vi "Finish.vi"   [LabVIEW 2014]
doc: "This VI is called just before exiting. It is expected to close I/O refnum, save collected data, etc."
uses:
  <vilib>/Rock Robotics/WPI/Joystick/WPI_JoystickGetSetRefNum.vi
  <vilib>/Rock Robotics/WPI/RobotDrive/WPI_RobotDriveGetSetRefNum.vi
types:
  T1 = typedef "WPI_RobotDriveDevRef.ctl" = cluster{"DevStatus":errorcluster, "Motors[]":T2[], "Square Inputs":bool, "Max Output":dbl}
  T2 = typedef "WPI_MotorControlDeviceRef.ctl" = cluster{"DeviceStatus":errorcluster, "Type":T3, "PWM":cluster{"Controller":T4, "PWM Channel":T5, "DeadBand":T6}, "CAN":cluster{"Device Number":u8, "Control Mode":T7, "Semaphore":T8, "Max Vout":dbl, "TalonSRX Control Mode":T9}, "Invert":bool, "TransformRef":T10, "InvTransformRef":T10}
  T3 = typedef "WPI_MotorControlType.ctl" = enum16{"PWM", "CAN", "CANTalonSRX"}
  T4 = typedef "FPGA_TypedefDigitalModule.ctl" = enum16{"Controller 1"}
  T5 = typedef "FPGA_DIOPWMChannel.ctl" = enum8{"PWM 0", "PWM 1", "PWM 2", "PWM 3", "PWM 4", "PWM 5", "PWM 6", "PWM 7", "PWM 8", "PWM 9", "PWM MXP 0", "PWM MXP 1", "PWM MXP 2", "PWM MXP 3", "PWM MXP 4", "PWM MXP 5", "PWM MXP 6", "PWM MXP 7", "PWM MXP 8", "PWM MXP 9", "Invalid"}
  T6 = typedef "WPI_PWMDeadband.ctl" = cluster{"Name":string, "maxPositivePwm":i32, "minPositivePwm":i32, "centerPwm":i32, "maxNegativePwm":i32, "minNegativePwm":i32, "angularRange":u16}
  T7 = typedef "WPI_CANJaguar_ControlMode.ctl" = enum8{"Percent VBus", "Current", "Speed", "Position", "Voltage"}
  T8 = typedef "Semaphore RefNum" = refnum<k1>
  T9 = typedef "WPI_CANTalonSRX_APIControlMode.ctl" = enum8{"Percent VBus", "Speed", "Position", "Slave", "Unchanged / Invalid"}
  T10 = typedef "WPI_PWMTransform_ConPane.ctl" = refnum<vi>
  T11 = typedef "WPI_JoystickDevRef.ctl" = cluster{"Device":T12}
  T12 = typedef "WPI_JoystickDeviceEnum.ctl" = enum16{"USB 0", "USB 1", "USB 2", "USB 3", "USB 4", "USB 5"}
  T13 = typedef "WPI_EncoderDevRef.ctl" = cluster{"DevStatus":errorcluster, "EncoderIndex":T14, "CounterIndex":T15, "DistancePerCount":dbl, "Decoding Type":T16}
  T14 = typedef "FPGA_EncoderIdx.ctl" = enum8{"Enc 0", "Enc 1", "Enc 2", "Enc 3", "Enc 4", "Enc 5", "Enc 6", "Enc 7", "Invalid"}
  T15 = typedef "FPGA_CounterCtrSystemIndex.ctl" = enum8{"Ctr 0", "Ctr 1", "Ctr 2", "Ctr 3", "Ctr 4", "Ctr 5", "Ctr 6", "Ctr 7", "Invalid"}
  T16 = typedef "WPI_EncoderType.ctl" = enum16{"1x", "2x", "4x"}
  T17 = typedef "WPI_SolenoidDevRef.ctl" = cluster{"DevStatus":errorcluster, "Pneumatics Control Module":u8, "Forward Solenoid Channel":T18, "Reverse Solenoid Channel":T18}
  T18 = typedef "WPI_SolenoidChannel.ctl" = enum8{"Solenoid 0", "Solenoid 1", "Solenoid 2", "Solenoid 3", "Solenoid 4", "Solenoid 5", "Solenoid 6", "Solenoid 7", "Invalid"}
  T19 = typedef "WPI_PotentiometerDevRef.ctl" = cluster{"DevStatus":errorcluster, "Controller":T20, "Analog Channel":T21, "Invert Output":bool}
  T20 = typedef "FPGA_TypedefAnalogModule.ctl" = enum16{"Controller 1"}
  T21 = typedef "FPGA_AIChannel.ctl" = enum8{"AI 0", "AI 1", "AI 2", "AI 3", "AI MXP 0", "AI MXP 1", "AI MXP 2", "AI MXP 3", "Invalid"}
  T22 = typedef "WPI_DigitalInputDevRef.ctl" = cluster{"DevStatus":errorcluster, "DIO Channel":T23, "Controller":T4}
  T23 = typedef "FPGA_DIOChannel.ctl" = enum8{"DIO 0", "DIO 1", "DIO 2", "DIO 3", "DIO 4", "DIO 5", "DIO 6", "DIO 7", "DIO 8", "DIO 9", "DIO MXP 0", "DIO MXP 1", "DIO MXP 2", "DIO MXP 3", "DIO MXP 4", "DIO MXP 5", "DIO MXP 6", "DIO MXP 7", "DIO MXP 8", "DIO MXP 9", "DIO MXP 10", "DIO MXP 11", "DIO MXP 12", "DIO MXP 13", "DIO MXP 14", "DIO MXP 15", "Invalid"}
  T24 = typedef "WPI_GyroDevRef.ctl" = cluster{"DevStatus":errorcluster, "Analog Module":T20, "Analog Channel":T21, "Offset":dbl, "Gain (VoltsPerDegree/Second)":dbl}
  T25 = typedef "WPI_I2CDevRef.ctl" = cluster{"DevStatus":errorcluster, "Controller":T4, "Device Address":u8, "Handle":i32, "I2C Bus":T26}
  T26 = typedef "i2c_bus.ctl" = enum16{"I2C On-Board", "I2C MXP", "Invalid"}
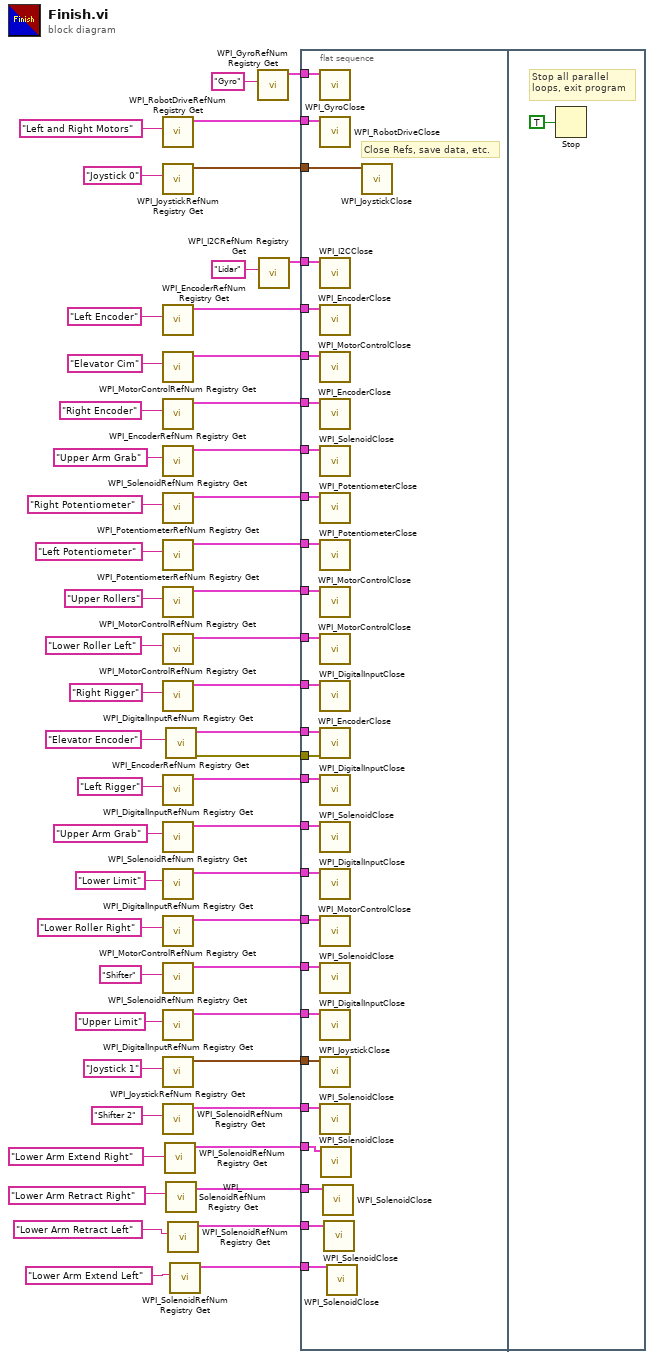
[diagram p0: block diagram]
diagram:
  n1 = call <vilib>:"WPI_RobotDriveRefNum Registry Get.vi"("refnum name"="Left and Right Motors") -> ("RobotDriveDevRef"=w51:T1)  [unwired: 1 in, 9 out]
  n2 = call <vilib>:"WPI_JoystickRefNum Registry Get.vi"("refnum name"="Joystick 0") -> ("JoystickDevRef"=w50:T11)  [unwired: 1 in, 9 out]
  n3 = call <vilib>:"WPI_EncoderRefNum Registry Get.vi"("refnum name"="Left Encoder") -> ("EncoderDevRef"=w14:T13)  [unwired: 9 in, 1 out]
  n4 = call <vilib>:"WPI_MotorControlRefNum Registry Get.vi"("refnum name"="Elevator Cim") -> ("MotorControlDevRef"=w48:T2)  [unwired: 9 in, 1 out]
  n5 = call <vilib>:"WPI_EncoderRefNum Registry Get.vi"("refnum name"="Right Encoder") -> ("EncoderDevRef"=w13:T13)  [unwired: 9 in, 1 out]
  n6 = call <vilib>:"WPI_SolenoidRefNum Registry Get.vi"("refnum name"="Upper Arm Grab") -> ("SolenoidDevRef"=w47:T17)  [unwired: 9 in, 1 out]
  n7 = call <vilib>:"WPI_PotentiometerRefNum Registry Get.vi"("refnum name"="Right Potentiometer") -> ("PotDevRef"=w17:T19)  [unwired: 9 in, 1 out]
  n8 = call <vilib>:"WPI_PotentiometerRefNum Registry Get.vi"("refnum name"="Left Potentiometer") -> ("PotDevRef"=w18:T19)  [unwired: 9 in, 1 out]
  n9 = call <vilib>:"WPI_MotorControlRefNum Registry Get.vi"("refnum name"="Upper Rollers") -> ("MotorControlDevRef"=w26:T2)  [unwired: 9 in, 1 out]
  n10 = call <vilib>:"WPI_MotorControlRefNum Registry Get.vi"("refnum name"="Lower Roller Left") -> ("MotorControlDevRef"=w20:T2)  [unwired: 9 in, 1 out]
  n11 = call <vilib>:"WPI_DigitalInputRefNum Registry Get.vi"("refnum name"="Right Rigger") -> ("DigitalInputDevRef"=w27:T22)  [unwired: 9 in, 1 out]
  n12 = call <vilib>:"WPI_DigitalInputRefNum Registry Get.vi"("refnum name"="Left Rigger") -> ("DigitalInputDevRef"=w28:T22)  [unwired: 9 in, 1 out]
  n13 = call <vilib>:"WPI_SolenoidRefNum Registry Get.vi"("refnum name"="Upper Arm Grab") -> ("SolenoidDevRef"=w40:T17)  [unwired: 9 in, 1 out]
  n14 = call <vilib>:"WPI_DigitalInputRefNum Registry Get.vi"("refnum name"="Lower Limit") -> ("DigitalInputDevRef"=w36:T22)  [unwired: 9 in, 1 out]
  n15 = call <vilib>:"WPI_MotorControlRefNum Registry Get.vi"("refnum name"="Lower Roller Right") -> ("MotorControlDevRef"=w22:T2)  [unwired: 9 in, 1 out]
  n16 = call <vilib>:"WPI_SolenoidRefNum Registry Get.vi"("refnum name"="Shifter") -> ("SolenoidDevRef"=w44:T17)  [unwired: 9 in, 1 out]
  n17 = call <vilib>:"WPI_DigitalInputRefNum Registry Get.vi"("refnum name"="Upper Limit") -> ("DigitalInputDevRef"=w37:T22)  [unwired: 9 in, 1 out]
  n18 = call <vilib>:"WPI_JoystickRefNum Registry Get.vi"("refnum name"="Joystick 1") -> ("JoystickDevRef"=w38:T11)  [unwired: 1 in, 9 out]
  n19 = call <vilib>:"WPI_SolenoidRefNum Registry Get.vi"("refnum name"="Shifter 2") -> ("SolenoidDevRef"=w42:T17)  [unwired: 9 in, 1 out]
  n20 = call <vilib>:"WPI_SolenoidRefNum Registry Get.vi"("refnum name"="Lower Arm Extend Right") -> ("SolenoidDevRef"=w8:T17)  [unwired: 9 in, 1 out]
  n21 = call <vilib>:"WPI_EncoderRefNum Registry Get.vi"("refnum name"="Elevator Encoder") -> ("error out"=w32:errorcluster, "EncoderDevRef"=w33:T13)  [unwired: 9 in]
  n22 = call <vilib>:"WPI_SolenoidRefNum Registry Get.vi"("refnum name"="Lower Arm Retract Right") -> ("SolenoidDevRef"=w7:T17)  [unwired: 9 in, 1 out]
  n23 = call <vilib>:"WPI_SolenoidRefNum Registry Get.vi"("refnum name"="Lower Arm Retract Left") -> ("SolenoidDevRef"=w2:T17)  [unwired: 9 in, 1 out]
  n24 = call <vilib>:"WPI_SolenoidRefNum Registry Get.vi"("refnum name"="Lower Arm Extend Left") -> ("SolenoidDevRef"=w1:T17)  [unwired: 9 in, 1 out]
  n25 = call <vilib>:"WPI_GyroRefNum Registry Get.vi"("refnum name"="Gyro") -> ("GyroDevRef"=w10:T24)  [unwired: 9 in, 1 out]
  n26 = call <vilib>:"WPI_I2CRefNum Registry Get.vi"("refnum name"="Lidar") -> ("I2CDevRef"=w24:T25)  [unwired: 9 in, 1 out]
  n27 = flat-sequence {
    tunnel: w51 -> [w80]
    tunnel: w50 -> [w79]
    tunnel: w48 -> [w78]
    tunnel: w47 -> [w73]
    tunnel: w44 -> [w77]
    tunnel: w42 -> [w76]
    tunnel: w40 -> [w75]
    tunnel: w38 -> [w74]
    tunnel: w37 -> [w72]
    tunnel: w36 -> [w71]
    tunnel: w33 -> [w70]
    tunnel: w32 -> [w69]
    tunnel: w28 -> [w68]
    tunnel: w27 -> [w67]
    tunnel: w26 -> [w66]
    tunnel: w24 -> [w65]
    tunnel: w22 -> [w64]
    tunnel: w20 -> [w63]
    tunnel: w18 -> [w62]
    tunnel: w17 -> [w61]
    tunnel: w14 -> [w60]
    tunnel: w13 -> [w59]
    tunnel: w10 -> [w58]
    tunnel: w8 -> [w57]
    tunnel: w7 -> [w56]
    tunnel: w2 -> [w55]
    tunnel: w1 -> [w54]
    frame #0 {
      # "Close Refs, save data, etc."
      n28 = call <vilib>:"WPI_GyroClose.vi"("GyroDevRef"=w58) -> ()  [unwired: 10 in, 1 out]
      n29 = call <vilib>:"WPI_RobotDriveClose.vi"("RobotDriveDevRef"=w80) -> ()  [unwired: 1 in, 10 out]
      n30 = call <vilib>:"WPI_I2CClose.vi"("I2CDevRef"=w65) -> ()  [unwired: 10 in, 1 out]
      n31 = call <vilib>:"WPI_EncoderClose.vi"("EncoderDevRef"=w60) -> ()  [unwired: 10 in, 1 out]
      n32 = call <vilib>:"WPI_MotorControlClose.vi"("MotorControlDevRef"=w78) -> ()  [unwired: 10 in, 1 out]
      n33 = call <vilib>:"WPI_EncoderClose.vi"("EncoderDevRef"=w59) -> ()  [unwired: 10 in, 1 out]
      n34 = call <vilib>:"WPI_SolenoidClose.vi"("SolenoidDevRef"=w73) -> ()  [unwired: 10 in, 1 out]
      n35 = call <vilib>:"WPI_PotentiometerClose.vi"("PotDevRef"=w61) -> ()  [unwired: 10 in, 1 out]
      n36 = call <vilib>:"WPI_PotentiometerClose.vi"("PotDevRef"=w62) -> ()  [unwired: 10 in, 1 out]
      n37 = call <vilib>:"WPI_MotorControlClose.vi"("MotorControlDevRef"=w66) -> ()  [unwired: 10 in, 1 out]
      n38 = call <vilib>:"WPI_MotorControlClose.vi"("MotorControlDevRef"=w63) -> ()  [unwired: 10 in, 1 out]
      n39 = call <vilib>:"WPI_DigitalInputClose.vi"("DigitalInputDevRef"=w67) -> ()  [unwired: 10 in, 1 out]
      n40 = call <vilib>:"WPI_EncoderClose.vi"("error in (no error)"=w69, "EncoderDevRef"=w70) -> ()  [unwired: 9 in, 1 out]
      n41 = call <vilib>:"WPI_DigitalInputClose.vi"("DigitalInputDevRef"=w68) -> ()  [unwired: 10 in, 1 out]
      n42 = call <vilib>:"WPI_SolenoidClose.vi"("SolenoidDevRef"=w75) -> ()  [unwired: 10 in, 1 out]
      n43 = call <vilib>:"WPI_DigitalInputClose.vi"("DigitalInputDevRef"=w71) -> ()  [unwired: 10 in, 1 out]
      n44 = call <vilib>:"WPI_MotorControlClose.vi"("MotorControlDevRef"=w64) -> ()  [unwired: 10 in, 1 out]
      n45 = call <vilib>:"WPI_SolenoidClose.vi"("SolenoidDevRef"=w77) -> ()  [unwired: 10 in, 1 out]
      n46 = call <vilib>:"WPI_DigitalInputClose.vi"("DigitalInputDevRef"=w72) -> ()  [unwired: 10 in, 1 out]
      n47 = call <vilib>:"WPI_JoystickClose.vi"("JoystickDevRef"=w74) -> ()  [unwired: 11 out]
      n48 = call <vilib>:"WPI_SolenoidClose.vi"("SolenoidDevRef"=w76) -> ()  [unwired: 10 in, 1 out]
      n49 = call <vilib>:"WPI_SolenoidClose.vi"("SolenoidDevRef"=w57) -> ()  [unwired: 10 in, 1 out]
      n50 = call <vilib>:"WPI_SolenoidClose.vi"("SolenoidDevRef"=w56) -> ()  [unwired: 10 in, 1 out]
      n51 = call <vilib>:"WPI_SolenoidClose.vi"("SolenoidDevRef"=w55) -> ()  [unwired: 10 in, 1 out]
      n52 = call <vilib>:"WPI_SolenoidClose.vi"("SolenoidDevRef"=w54) -> ()  [unwired: 10 in, 1 out]
      n53 = call <vilib>:"WPI_JoystickClose.vi"("JoystickDevRef"=w79) -> ()  [unwired: 11 out]
    }
    frame #1 {
      # "Stop all parallel\nloops, exit program"
      n54 = Stop(stop? (T)=TRUE ("Quit")) -> ()
    }
  }
